vi "Exp CDF.vi"(9 "b":dbl=3.0, 10 "a":dbl=1.0, 11 "x":dbl=3.0) -> (0 "error":i32, 3 "cdf(x)":dbl=0.486582880967408)   [LabVIEW 2020, in "NI_Gmath.lvlib"]
doc: "Computes the continuous cumulative distribution function (CDF), or the probability that the random variate X, where X describes the selected distribution type, has a value less than or equal to <B>x</B>. You must manually select the polymorphic instance to use."
uses:
  <vilib>/gmath/NI_Gmath.lvlib
  <vilib>/gmath/statdist.llb/st_error_code.ctl
panel:
  # "Exp CDF"
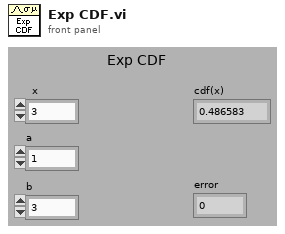
[diagram p1: front panel]
types:
  T1 = typedef "NI_Gmath.lvlib/st_error_code.ctl" = i32
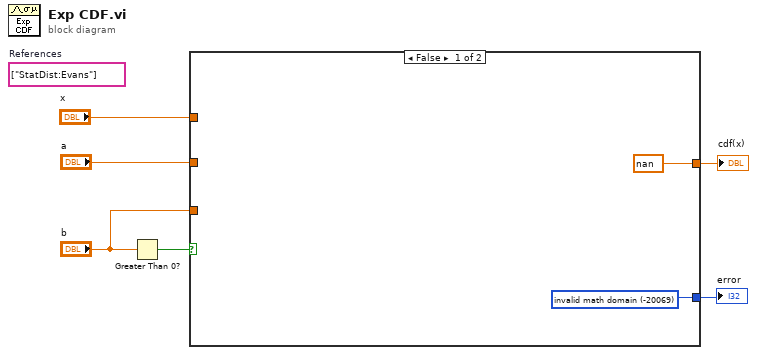
[diagram p0: block diagram]
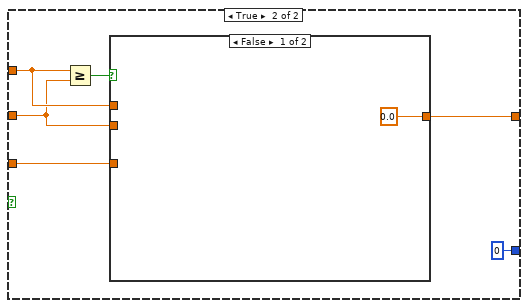
[diagram p2: hidden frame]
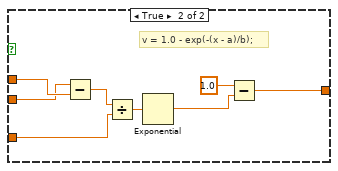
[diagram p3: hidden frame]
diagram:
  (unwired) string[] ["StatDist:Evans"]  # References
  n1 = Greater Than 0?(x="b") -> (x > 0?=w2:bool)
  n2 = case shown="False" w2 {
    tunnel: "b" -> [_ w12]
    tunnel: [w7 0 ("invalid math domain")] -> w6
    tunnel: [nan w13] -> w5
    tunnel: "x" -> [_ w10]
    tunnel: "a" -> [_ w9]
    frame False {
      w7 = T1 -20069 items=["invalid math domain"=-20069, "Fourier interpolation size m >= n"=-20070, "empty array"=-20003] ("stat interp error code")
    }
    frame True {
      n3 = Greater Or Equal?(x=w10, y=w9) -> (x >= y?=w11:bool)
      n4 = case shown="False" w11 {
        tunnel: [0.0 w16] -> w13
        tunnel: w10 -> [_ w23]
        tunnel: w9 -> [_ w22]
        tunnel: w12 -> [_ w19]
        frame False {
        }
        frame True {
          # "v = 1.0 - exp(-(x - a)/b);"
          n5 = Subtract(x=w22, y=w23) -> (x-y=w21:dbl)
          n6 = Divide(x=w21, y=w19) -> (x/y=w20:dbl)
          n7 = Exponential(1:w20) -> (0:w17:dbl)
          n8 = Subtract(x=1.0, y=w17) -> (x-y=w16:dbl)
        }
      }
    }
  }
  "cdf(x)" <- w5
  "error" <- w6
